vi "Intan_StreamData_128ch_parallelLoop.vi"(0 "VISA resource name":refnum<visa-resource-name>, 1 "refnum in":refnum<file>, 2 "NchansInStream":u16, 3 "stop streaming":bool, 4 "Save Binary Data":bool, 5 "error in":errorcluster, 7 "byte order":T5(ring)=enum."little-endian", 8 "hdr fpath":path, 9 "MaxStreamChans":u16=32, 11 "DT_scale (sec)":dbl=0.01, 12 "aux file ref num":refnum<file>, 14 "save aux file":bool) -> (6 "N data scans to read (VISA)":i32=20, 10 "Nbytes VISA read":u32, 13 "VISA read iter":i32, 19 "error out":errorcluster)   [LabVIEW 2017]
doc: "Stream data to disk and user friendly display. Data is scaled and filtered prior to display.\n\nThis VI uses parallel while loop architecture: 1 loop reads from serial stream and saves raw bytes to disk; the other loop processes the data in chunk, scaling and filtering, then displays."
uses:
  zip_swcircularbuffer1_0_19b/Circular Buffer/Controls/Circular Buffer Status.ctl
  zip_swcircularbuffer1_0_19b/Circular Buffer/Controls/Circular Buffer Operations.ctl
  <vilib>/Utility/error.llb/DialogType.ctl
  zip_swcircularbuffer1_0_19b/Circular Buffer/Instance VIs/Circular Buffer(1D U16).vi
  zip_swcircularbuffer1_0_19b/Circular Buffer/Circular Buffer.lvlib
panel:
  out "bytesParsed":i32=148
  out "Buffer Status Empty Buf":T1
  out "termcharsReadBuffer":string
  out "termcharsCount":u32
  out "NumChansNewStream":string
  out "Data Out":u16[](array[numeric])
  out "Elements Remaining":i32
  out "ChanSelString":string
  out "ChanSelect(uint32)":u32[](array[numeric])
  out "A+B+C+D chans":i32[](array[numeric])
  out "C+D chans":i32[](array[numeric])
  out "Dchans":i32[](array[numeric])
  out "Cchans":i32[](array[numeric])
  out "ADXL Stream":dbl[][](graph)
  out "A+B chans":i32[](array[numeric])
  out "Bchans":i32[](array[numeric])
  out "Achans":i32[](array[numeric])
  in  "Tab Control":T2(tab)
  in  "Update Channels":bool
  in  "Accel/Vbat":i32[](listbox)
  in  "stop logging":bool
  in  "DisplayScale (uV/div)":u16(ring)=1 items=["6400", "3200", "1600", "800", "400", "200", "100", "50", "25"]
  in  "offset factor":dbl=1.0
  in  "Filter settings":T3={"LP Filter On/Off"=TRUE, "LP Cutoff (Hz)"=40.0, "HP Filter On/Off"=TRUE, "HP Cutoff (Hz)"=0.5, "Bandstop On/Off"=TRUE, "fl Cutoff (Hz)"=48.0, "fh Cutoff (Hz) "=52.0}
  out "Save status":bool
  out "non integer read":bool
  out "display iter":i32
  out "% buffer full":dbl(slide) scale=0.0..100.0
  in  "Ring Buffer Size":T4={"Samples per Channel"=640000, "Channels"=0}
  out "buffer underflow":bool
  out "Buffer Status  (read)":T1
  out "buffer overflow":bool
  out "Buffer Status (write)":T1
  in  "Center Traces":bool
  in  "Amplifier Chans":i32[](listbox)=[1, 4, 13, 14, 15, 16, 17, 22]
  out "FS (Hz)":dbl
  in  "ChartDisplayLength (s)":dbl=5.0
  in  "Display Update interval (ms)":dbl=100.0
  in  "Buffer Read Interval (ms)":dbl=100.0
  in  "ChanSelect":u16(ring) items=["A chans (0-31)", "B chans (32-63)", "C chans (64-95)", "D chans (96-127)", "Free Select"]
  in  "bytes per data frame":i32=286
  in  "Nchans":i32=128
  in  "start stream (Teensy char)":string="s"
  in  "stop serial stream (Teensy char)":string="t"
  out "Text response":string
  out "timestamp_array":i32[](array[numeric])
  out "aux_cmd_array":i32[][](array[numeric])
  out "binary data (from VISA read)":u16[](array[numeric])
  out "magicNum Out":i32[](array[numeric])
  in  "stop logging Teensy char":string="l"
  out "Vdd (V) out":dbl[](array[numeric])
  out "setscaleresult":dbl
  out "UpdateCode":i16
  out "xmax_init":dbl
  out "offset_init":dbl
  out "increment_init":dbl
  out "xmin_init":dbl
  out "NchansChanged":bool
  out "DispLengthChanged":bool
  out "XscaleRollover":bool
  out "error code out":i32 format="%0.0f"
  out "StopLoopsMaster":bool
  out "N_u16s  write to buf":i32
  out "Nelements to read from buf":dbl
  out "N data scans to display":u16=20
  out "YtxtLabelsAll":string[](array[string])
  out "bytes streaming per frame":u16
  out "requestBytes":dbl
  out "SerRead":string
  out "Picture":picture
  out "Intan Streaming Data":dbl[][](graph)
  # "Intan-Teensy Bioelectric Module: Data Stream and Visualization\n128 chan + ADXL"
  # "Data Streaming Frequency"
  # "Display Settings"
  # "Ring Buffer Status"
  # "1-D data stream \nreformatted  to 2-D"
  # "xscale controls"
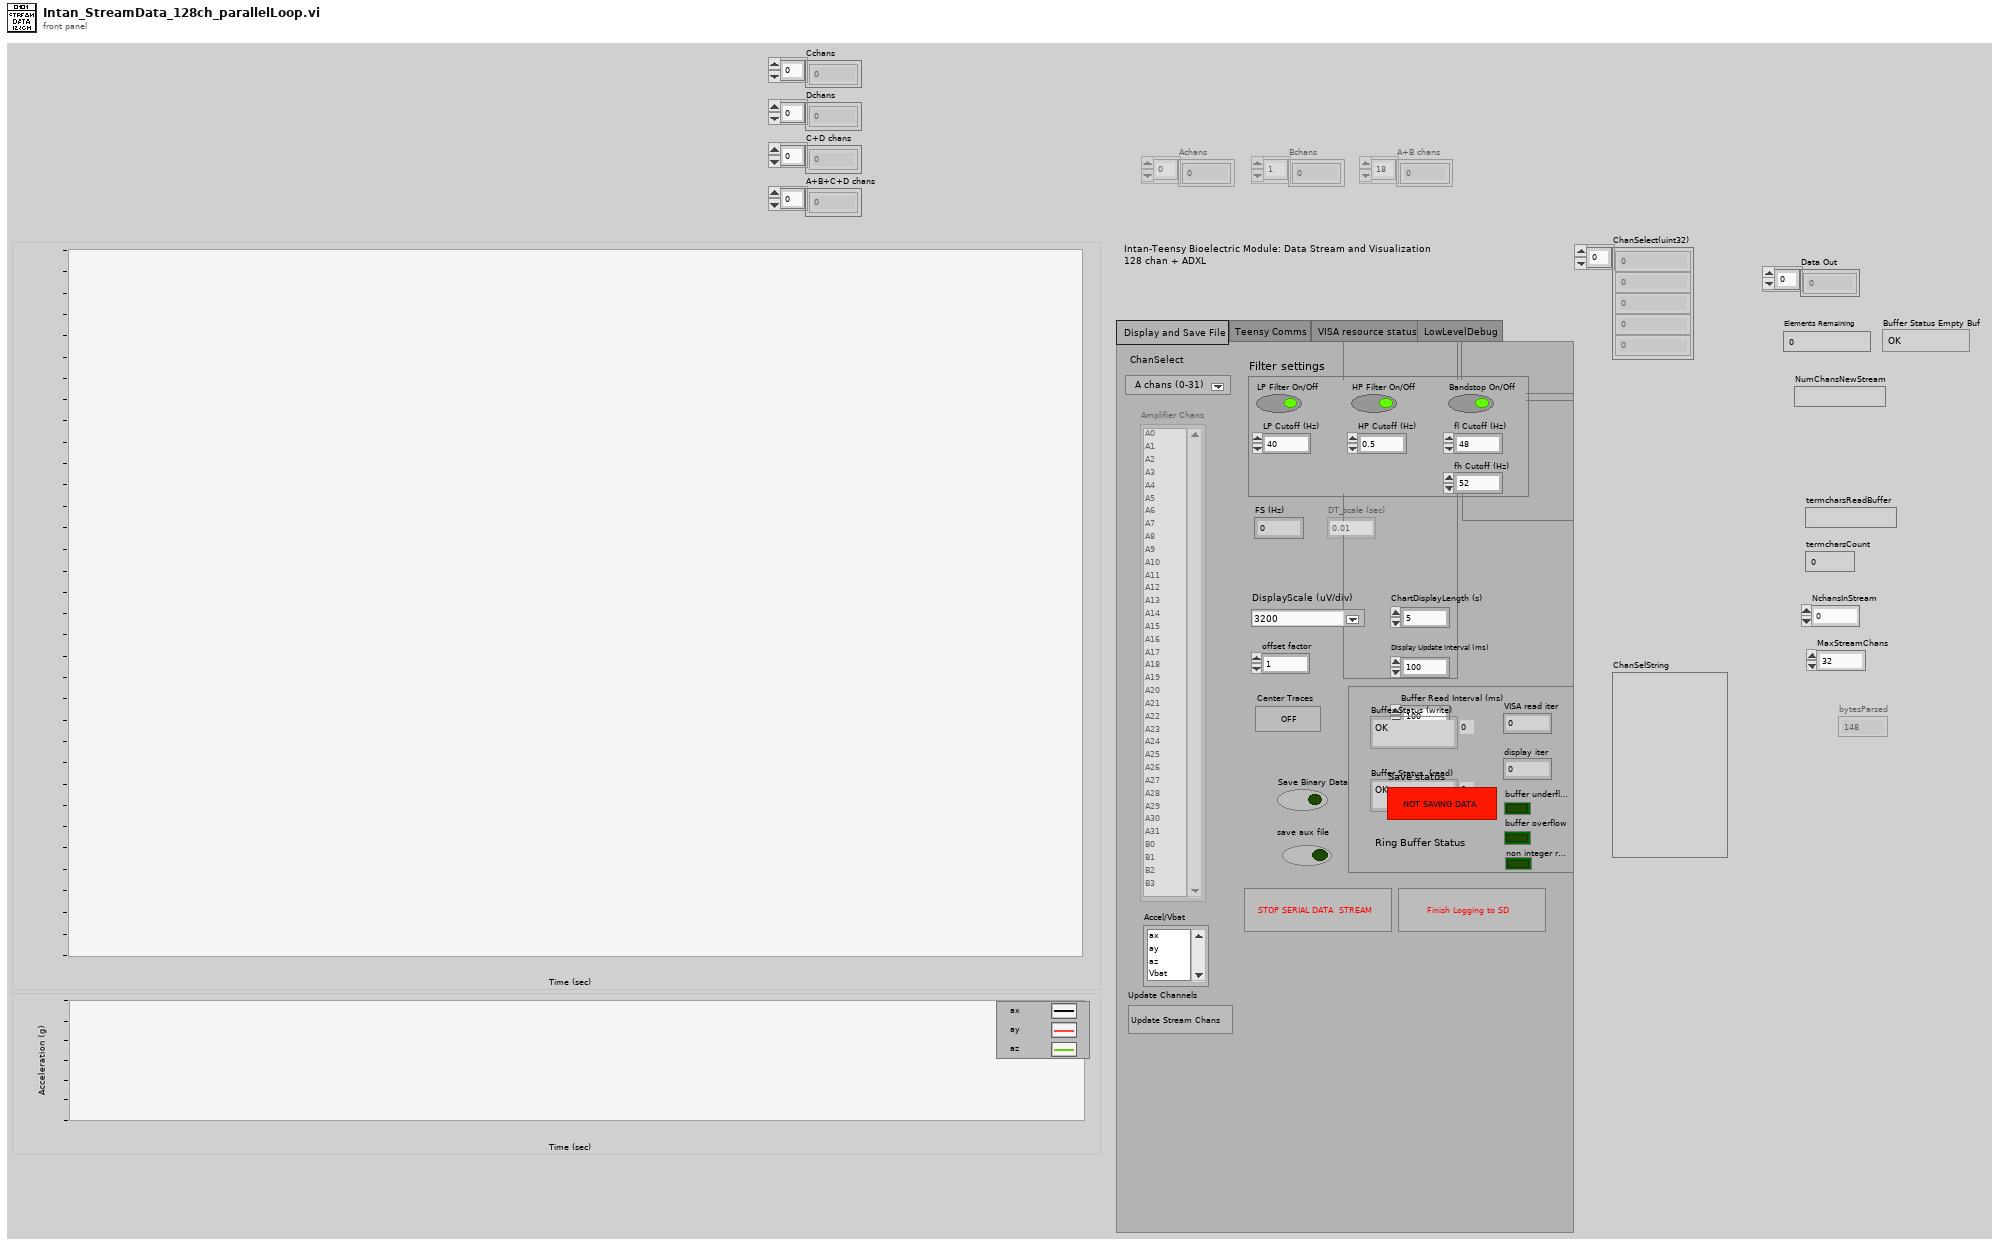
[diagram p1: front panel]
types:
  T1 = typedef "Circular Buffer.lvlib/Circular Buffer Status.ctl" = enum16{"OK", "Overflow", "Underflow"}
  T2 = enum32{"Display and Save File ", "Teensy Comms", "VISA resource status", "LowLevelDebug"}
  T3 = cluster{"LP Filter On/Off":bool, "LP Cutoff (Hz)":dbl, "HP Filter On/Off":bool, "HP Cutoff (Hz)":dbl, "Bandstop On/Off":bool, "fl Cutoff (Hz)":dbl, "fh Cutoff (Hz) ":dbl}
  T4 = cluster{"Samples per Channel":u32, "Channels":u32}
  T5 = enum16{"big-endian, network order", "native, host order", "little-endian"}
  T6 = typedef "Circular Buffer.lvlib/Circular Buffer Operations.ctl" = enum16{"Initialize", "Get Backlog", "Write", "Read (continuous)", "Read (most recent)"}
  T7 = enum8{"Enabled", "Disabled", "Disabled and Grayed Out"}
  T8 = typedef "LVRectTypeDef.ctl" = cluster{"Left":i16, "Top":i16, "Right":i16, "Bottom":i16}
  T9 = cluster{"XScale.Minimum":dbl, "XScale.Maximum":dbl, "XScale.Increment":dbl, "Nchannels":i32}
  T10 = cluster{"Maximum":dbl, dbl, dbl, dbl, dbl, dbl, "YscleMark":dbl, "Increment":dbl}
  T11 = typedef "DialogType.ctl" = u16
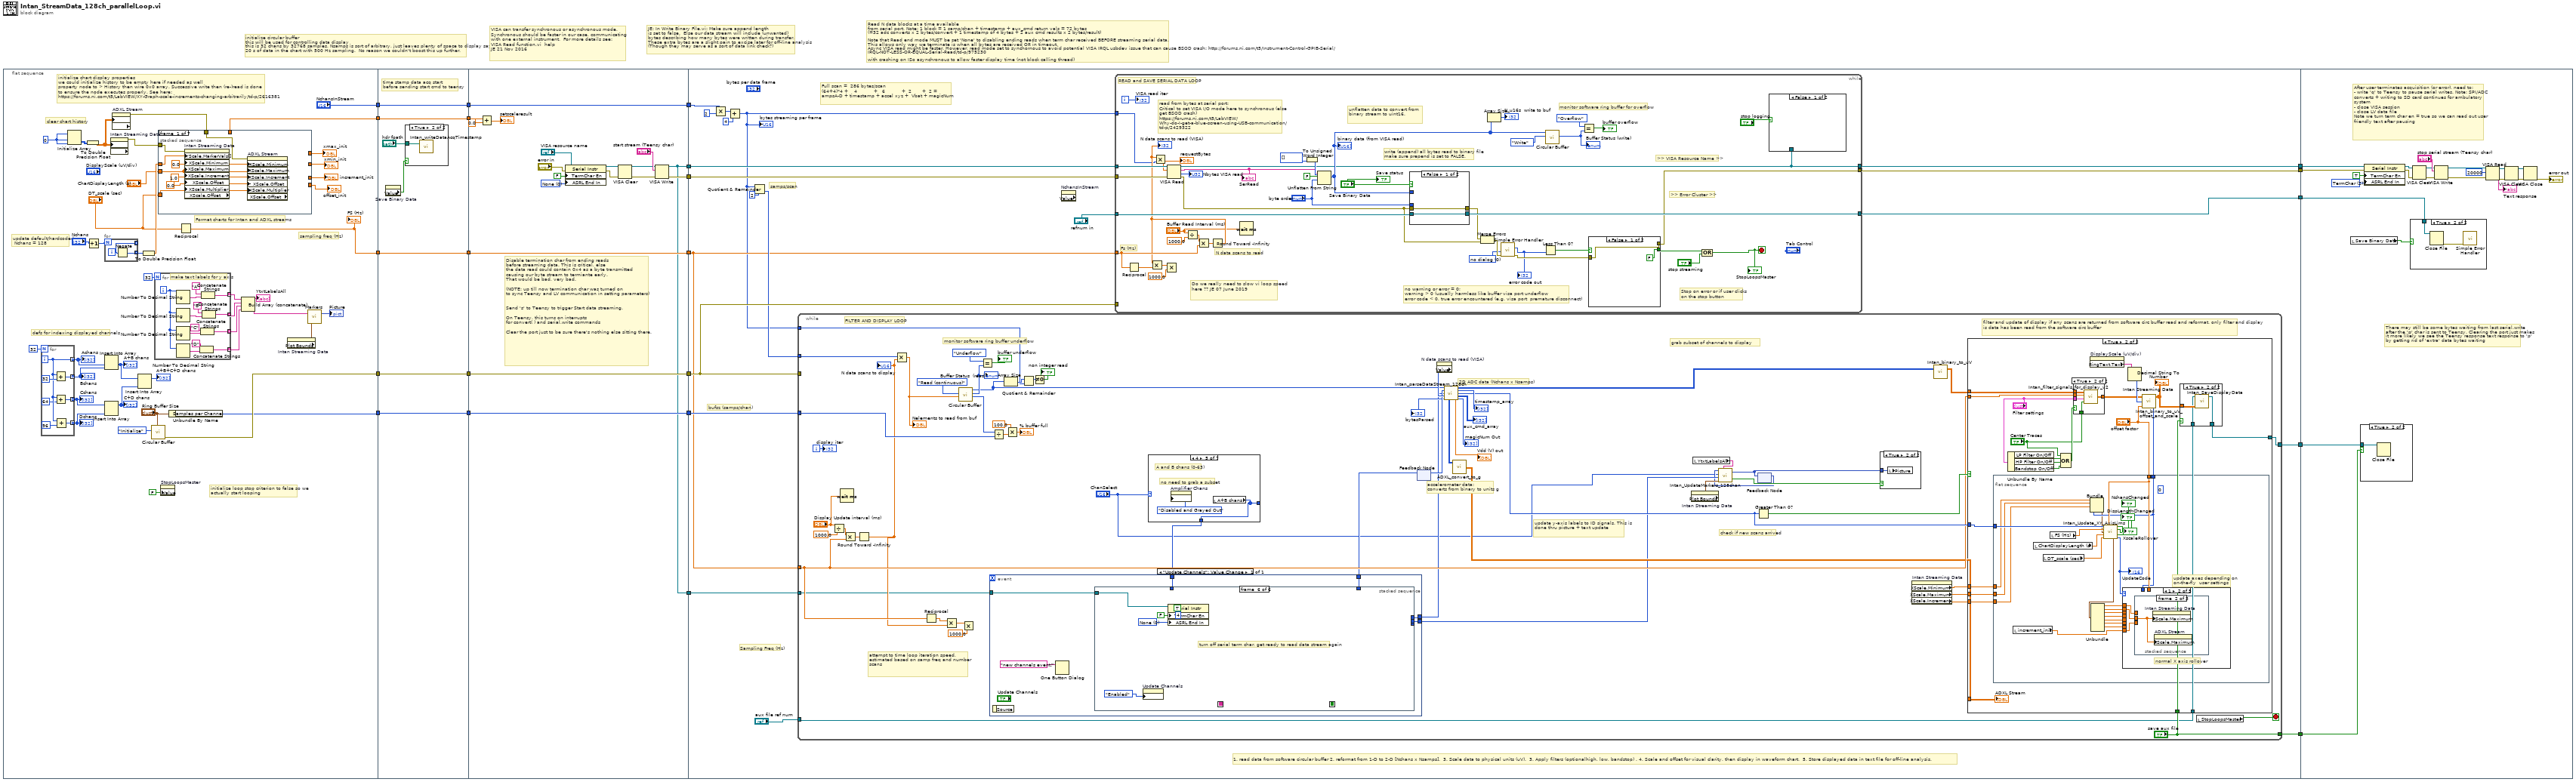
[diagram p0: block diagram]
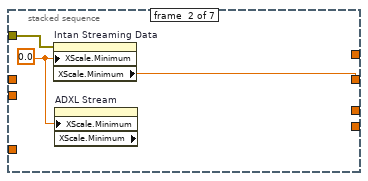
[diagram p2: hidden frame]
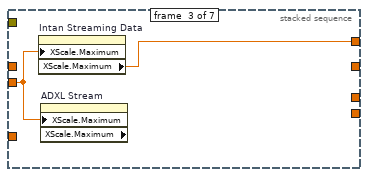
[diagram p3: hidden frame]
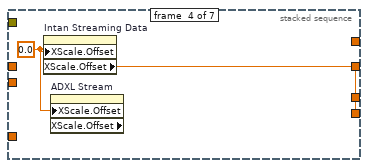
[diagram p4: hidden frame]
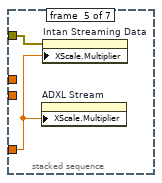
[diagram p5: hidden frame]
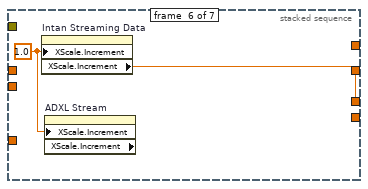
[diagram p6: hidden frame]
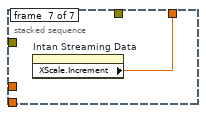
[diagram p7: hidden frame]
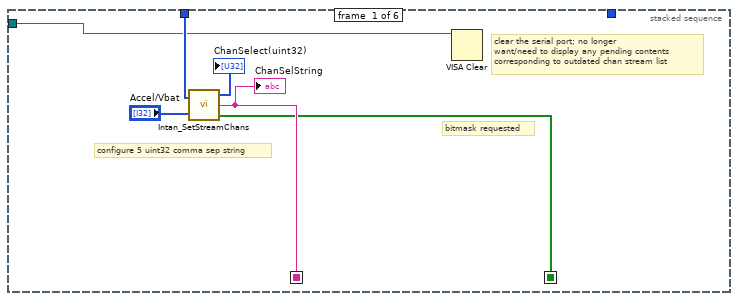
[diagram p9: hidden frame]
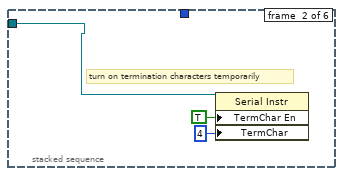
[diagram p10: hidden frame]
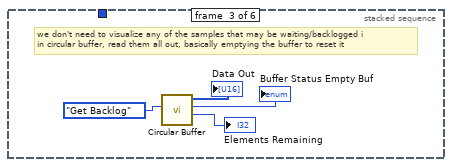
[diagram p11: hidden frame]
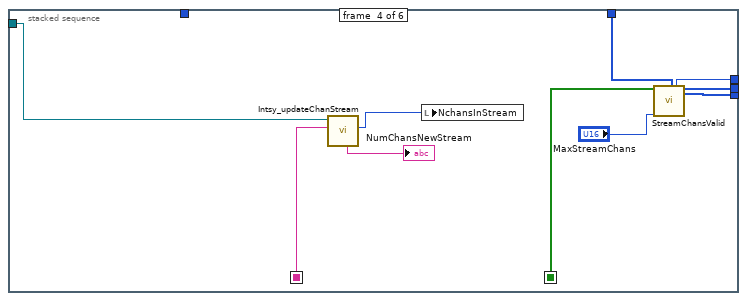
[diagram p12: hidden frame]
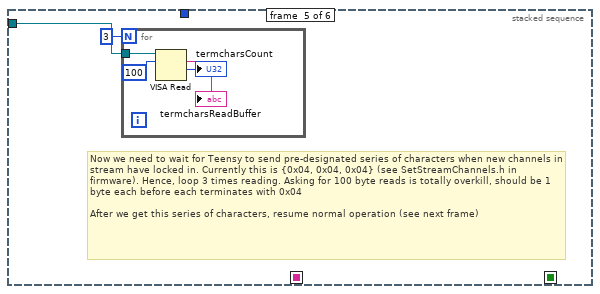
[diagram p13: hidden frame]
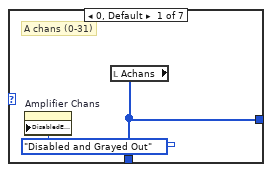
[diagram p15: hidden frame]
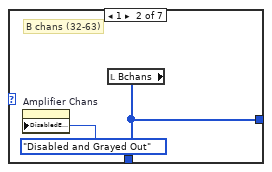
[diagram p16: hidden frame]
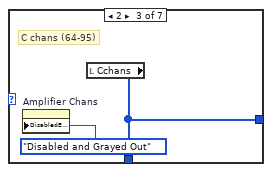
[diagram p17: hidden frame]
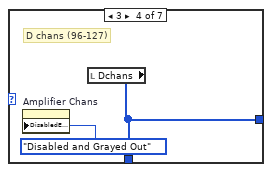
[diagram p18: hidden frame]
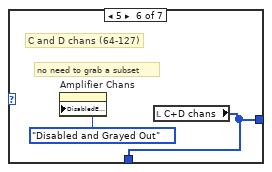
[diagram p19: hidden frame]
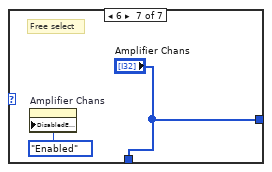
[diagram p20: hidden frame]
diagram:
  # "Read N data blocks at a time available\nfrom serial port. Note: 1 block = 1 samp/chan + timestamp + aux_cmd return vals = 72 bytes \n(=32 adc converts x 2 bytes/convert + 1 timestamp of 4 bytes + 2 aux cmd results x 2 bytes/result) \n\nNote that Read end mode MUST be set 'None' to disabling ending reads when term char received BEFORE streaming serial data.  \nThis allows only way we terminate is when all bytes are received OR in timeout.  \nAsync VISA read might be faster. However, read mode set to synchornous to avoid potential VISA IRQL usbdev issue that can cause BSOD crash: http://forums.ni.com/t5/Instrument-Control-GPIB-Serial/IRQL-NOT-LESS-OR-EQUAL-Serial-Read/td-p/975230\n\nwith crashing on ISo asynchronous to allow faster display time (not block calling thread)"
  # "initialize circular buffer\nthis will be used for controlling data display\nthis is 32 chans by 32768 samples. Nsamps is sort of arbitrary, just leaves plenty of space to display say\n20 s of data in the chart with 500 Hz sampling.  No reason we couldn't boost this up further."
  # "JE: In Write Binary File.vi: Make sure append length \nis set to false.  Else our data stream will include (unwanted)\nbytes describing how many bytes were written during transfer.\nThese extra bytes are a slight pain to excise later for off-line analysis\n(Though they may serve as a sort of data link check?)"
  # "VISA can transfer synchronous or asynchronous mode.\nSynchronous should be faster in our case, communicating\nwith one external instrument.  For more details see: \nVISA Read function.vi  help \nJE 21 Nov 2016"
  n1 = flat-sequence {
    tunnel: [w58] -> w12
    tunnel: [w56] -> w10
    tunnel: [w52] -> w8
    tunnel: [w41] -> w6
    tunnel: ["NchansInStream"] -> w3
    tunnel: w12 -> [w110]
    tunnel: [w110] -> w11
    tunnel: w10 -> [w109]
    tunnel: [w109] -> w9
    tunnel: w8 -> [w108]
    tunnel: [w108] -> w7
    tunnel: w6 -> [w107]
    tunnel: [w107] -> w5
    tunnel: w3 -> [w104]
    tunnel: [w104] -> w1
    tunnel: [w120] -> w20
    tunnel: [w113] -> w19
    tunnel: [w119] -> w18
    tunnel: w11 -> [w119]
    tunnel: [w118] -> w17
    tunnel: w9 -> [w118]
    tunnel: [w117] -> w16
    tunnel: w7 -> [w117]
    tunnel: w5 -> [w116]
    tunnel: [w113] -> w4
    tunnel: [w112] -> w2
    tunnel: w1 -> [w112]
    tunnel: [w145] -> w22
    tunnel: [w148] -> w21
    tunnel: w20 -> [w146]
    tunnel: w19 -> [w147]
    tunnel: w18 -> [w144]
    tunnel: w17 -> [w142]
    tunnel: w16 -> [w140]
    tunnel: [w139] -> w15
    tunnel: [w137] -> w14
    tunnel: [w136] -> w13
    tunnel: w4 -> [w135]
    tunnel: w2 -> [w134]
    tunnel: w22 -> [w425]
    tunnel: w21 -> [w438]
    tunnel: w15 -> [w420]
    tunnel: w14 -> [w419]
    tunnel: w13 -> [w418]
    frame #0 {
      w51 = 0 ("Dimension Size")
      # "Format charts for Intan and ADXL streams"
      # "defs for indexing displayed channels"
      # "update default/hardcoded\n Nchans = 128"
      # "clear chart history"
      # "initialize loop stop criterion to false so we\nactually start looping"
      # "sampling freq (Hz)"
      # "initialize chart display properties\nwe could initialize history to be empty here if needed as well\nproperty node to > History then wire 0x0 array. Successive write then (re-)read is done\nto ensure the node executes properly. See here:\nhttps://forums.ni.com/t5/LabVIEW/XY-Graph-scale-increments-changing-arbitrarily/td-p/2616381"
      n2 = for {
        N: 32 -> [_]
        tunnel: [w66] -> w33 mode=indexing
        tunnel: [w67] -> w32 mode=indexing
        tunnel: [w63] -> w31 mode=indexing
        tunnel: [w62] -> w30 mode=indexing
        i -> [w66]
        n3 = Add(x=w66, y=32) -> (x+y=w67:i32)
        n4 = Add(x=w66, y=64) -> (x+y=w63:i32)
        n5 = Add(x=w66, y=96) -> (x+y=w62:i32)
      }
      "Achans" <- w33
      "Bchans" <- w32
      "Cchans" <- w31
      "Dchans" <- w30
      n6 = Initialize Array(w51, w51, w51) -> (w50:i32[][])
      n7 = To Double Precision Float(number=w50) -> (double precision float=w35:dbl[][])
      n8 = Increment(x="Nchans") -> (x+1=w60:i32)
      n9 = for {
        N: w60 -> [_]
        tunnel: [w103] -> w61 mode=indexing
        tunnel: [w102] -> _ mode=indexing
        i -> [w102]
        n10 = Negate(x=w102) -> (-x=w103:i32)
      }
      n11 = Insert Into Array(array=w33, new element=w32) -> (w29:i32[])  [unwired: 1 in]
      "A+B chans" <- w29
      n12 = Insert Into Array(array=w31, new element=w30) -> (w28:i32[])  [unwired: 1 in]
      "C+D chans" <- w28
      n13 = property on="Intan Streaming Data" class="WFChart (strict)" props=["History Data", "History Data"]("History Data"=w35) -> (error out=w48:errorcluster)  [unwired: 2 in, 2 out]
      n14 = property on="ADXL Stream" class="WFChart (strict)" props=["History Data", "History Data"]("History Data"=w35) -> (error out=w34:errorcluster)  [unwired: 2 in, 2 out]
      n15 = Insert Into Array(array=w29, new element=w28) -> (→"A+B+C+D chans":i32[])  [unwired: 1 in]
      n16 = To Double Precision Float(number=w61) -> (double precision float=w49:dbl[])
      n17 = call-poly "Circular Buffer.vi"("Buffer Size"="Ring Buffer Size", "Operation"=Circular_Buffer_Operations."Initialize") -> ("error out"=w58:errorcluster)  [unwired: 6 in, 3 out]
      n18 = for {
        N: 32 -> [_]
        tunnel: [w99] -> w38 mode=indexing
        tunnel: [w96] -> w37 mode=indexing
        tunnel: [w90] -> w26 mode=indexing
        tunnel: [w89] -> w25 mode=indexing
        i -> [w95]
        # "make text labels for y axis"
        n19 = Number To Decimal String(number=w95) -> (decimal integer string=w101:string)  [unwired: 1 in]
        n20 = Number To Decimal String(number=w95) -> (decimal integer string=w98:string)  [unwired: 1 in]
        n21 = Number To Decimal String(number=w95) -> (decimal integer string=w91:string)  [unwired: 1 in]
        n22 = Number To Decimal String(number=w95) -> (decimal integer string=w92:string)  [unwired: 1 in]
        n23 = Concatenate Strings("D" ("string"), w92) -> (w89:string)
        n24 = Concatenate Strings("C" ("string"), w91) -> (w90:string)
        n25 = Concatenate Strings("A" ("string"), w101) -> (w99:string)
        n26 = Concatenate Strings("B" ("string"), w98) -> (w96:string)
      }
      n27 = stacked-sequence {
        tunnel: w49 -> [w76 _ _ _ _ _ _]
        tunnel: w48 -> [w75 w78 _ _ w85 _ _]
        tunnel: "ChartDisplayLength (s)" -> [w73 _ w80 _ _ _ _]
        tunnel: "DT_scale (sec)" -> [w70 _ _ _ w84 _ _]
        tunnel: [_ _ w81 _ _ _ _] -> w42
        tunnel: [_ w79 _ _ _ _ _] -> w45
        tunnel: [_ _ _ _ _ w87 _] -> w44
        tunnel: [_ _ _ w83 _ _ _] -> w43
        tunnel: [_ _ _ _ _ _ w88] -> w41
        tunnel: w34 -> [w69 _ _ _ _ _ _]
        frame #0 {
          w72 = 1.0 ("X Scale.Range:Minimum")
          w71 = 0.0 ("X Scale.Range:Minimum")
          w74 = 0.0 ("X Scale.Range:Minimum")
          n28 = property on="Intan Streaming Data" class="WFChart (strict)" props=["YScale", "MarkerVals[]", "XScale", "Minimum", "XScale", "Maximum", "XScale", "Increment", "XScale", "Offset", "XScale", "Multiplier", "XScale", "Offset"](error in=w75, "YScale.MarkerVals[]"=w76, "XScale.Minimum"=w74, "XScale.Maximum"=w73, "XScale.Increment"=w72, "XScale.Offset"=w71, "XScale.Multiplier"=w70) -> ()  [unwired: 1 in, 3 out]
          n29 = property on="ADXL Stream" class="WFChart (strict)" props=["XScale", "Minimum", "XScale", "Maximum", "XScale", "Increment", "XScale", "Offset", "XScale", "Multiplier", "XScale", "Offset"](error in=w69, "XScale.Minimum"=w74, "XScale.Maximum"=w73, "XScale.Increment"=w72, "XScale.Offset"=w71, "XScale.Multiplier"=w70) -> ()  [unwired: 1 in, 3 out]
        }
        frame #1 {
          w77 = 0.0 ("X Scale.Range:Minimum")
          n30 = property on="Intan Streaming Data" class="WFChart (strict)"(error in=w78, "XScale.Minimum"=w77) -> ("XScale.Minimum"=w79:dbl)  [unwired: 1 in, 2 out]
          n31 = property on="ADXL Stream" class="WFChart (strict)" props=["XScale", "Minimum", "XScale", "Minimum"]("XScale.Minimum"=w77) -> ()  [unwired: 2 in, 3 out]
        }
        frame #2 {
          n32 = property on="Intan Streaming Data" class="WFChart (strict)"("XScale.Maximum"=w80) -> ("XScale.Maximum"=w81:dbl)  [unwired: 2 in, 2 out]
          n33 = property on="ADXL Stream" class="WFChart (strict)" props=["XScale", "Maximum", "XScale", "Maximum"]("XScale.Maximum"=w80) -> ()  [unwired: 2 in, 3 out]
        }
        frame #3 {
          w82 = 0.0 ("X Scale.Offset and Multiplier:Offset")
          n34 = property on="Intan Streaming Data" class="WFChart (strict)"("XScale.Offset"=w82) -> ("XScale.Offset"=w83:dbl)  [unwired: 2 in, 2 out]
          n35 = property on="ADXL Stream" class="WFChart (strict)" props=["XScale", "Offset", "XScale", "Offset"]("XScale.Offset"=w82) -> ()  [unwired: 2 in, 3 out]
        }
        frame #4 {
          n36 = property on="ADXL Stream" class="WFChart (strict)"("XScale.Multiplier"=w84) -> ()  [unwired: 2 in, 2 out]
          n37 = property on="Intan Streaming Data" class="WFChart (strict)"(error in=w85, "XScale.Multiplier"=w84) -> ()  [unwired: 1 in, 2 out]
        }
        frame #5 {
          w86 = 1.0 ("X Scale.Range:Increment")
          n38 = property on="Intan Streaming Data" class="WFChart (strict)"("XScale.Increment"=w86) -> ("XScale.Increment"=w87:dbl)  [unwired: 2 in, 2 out]
          n39 = property on="ADXL Stream" class="WFChart (strict)" props=["XScale", "Increment", "XScale", "Increment"]("XScale.Increment"=w86) -> ()  [unwired: 2 in, 3 out]
        }
        frame #6 {
          n40 = property on="Intan Streaming Data" class="WFChart (strict)"() -> ("XScale.Increment"=w88:dbl)  [unwired: 2 in, 2 out]
        }
      }
      "xmin_init" <- w45
      "increment_init" <- w44
      "offset_init" <- w43
      "xmax_init" <- w42
      n41 = property on="StopLoopsMaster" class="Bool (strict)"("Value"=FALSE ("StopLoopsMaster")) -> ()  [unwired: 2 in, 2 out]
      n42 = Unbundle By Name("Ring Buffer Size") -> ("Samples per Channel"=w56:u32)
      n43 = Reciprocal(x="DT_scale (sec)") -> (1/x=w52:dbl)
      "FS (Hz)" <- w52
      n44 = Build Array (concatenate)(w38, w37, w26, w25) -> (w36:string[])
      "YtxtLabelsAll" <- w36
      n45 = property on="Intan Streaming Data" class="WFChart (strict)"() -> ("Plot Bounds"=w53:T8)  [unwired: 2 in, 2 out]
      n46 = call "Markers.vi"("plot bounds"=w53, "Array"=w36) -> ("Picture"=→"Picture":picture)  [unwired: 1 out]
    }
    frame #1 {
      # "time stamp data acq start\nbefore sending start cmd to teensy"
      n47 = property on="Save Binary Data" class="Bool (strict)"() -> ("Value"=w106:bool)  [unwired: 2 in, 2 out]
      n48 = case shown="True" w106 {
        tunnel: "hdr fpath" -> [_ w111]
        frame False {
        }
        frame True {
          n49 = call "Intan_writeDataAcqTimestamp.vi"("hdr fpath"=w111) -> ()  [unwired: 2 in, 1 out]
        }
      }
    }
    frame #2 {
      w125 = u16 0 items=["None", "Last Bit", "TermChar"] ("Serial Settings:End Mode for Reads")
      # "Disable termination char from ending reads\nbefore streaming data. This is critical, else\nthe data read could contain 0x4 as a byte transmitted\ncausing our byte stream to termiante early.\nThat would be bad, very bad.\n\n(NOTE: up till now termination char was turned on\nto sync Teensy and LV communication in setting parameters)\n\n\nSend 's' to Teensy to trigger Start data streaming.  \n\nOn Teensy, this turns on interrupts\nfor convert( ) and serial.write commands\n\nClear the port just to be sure there's nothing else sitting there."
      n50 = Add(x=w116, y=0.0) -> (x+y=→"setscaleresult":dbl)
      n51 = property class="Serial Instr"(reference="VISA resource name", error in="error in", "TermChar En"=FALSE ("Message Based Settings:Termination Character Enable"), "ASRL End In"=w125) -> (reference out=w124:refnum<visa-resource-name>, error out=w123:errorcluster)
      n52 = VISA Clear(VISA resource name=w124, error in (no error)=w123) -> (VISA resource name out=w122:refnum<visa-resource-name>, error out=w121:errorcluster)
      n53 = VISA Write(VISA resource name=w122, write buffer="start stream (Teensy char)", error in (no error)=w121) -> (VISA resource name out=w113:refnum<visa-resource-name>, error out=w120:errorcluster)  [unwired: 1 out]
    }
    frame #3 {
      # "Full scan =  286 bytes/scan\n(64+4)*4 +    4           +   6           +  2       +  2 =\nampsA-D + timestamp + accel xyz +  Vbat + magicNum"
      # "1. read data from software circular buffer 2. reformat from 1-D to 2-D [Nchans x Nsamps].  3. Scale data to physical units (uV).  3. Apply filters (optionalhigh, low, bandstop) . 4. Scale and offset for visual clarity, then display in waveform chart.  5. Store displayed data in text file for off-line analysis."
      # "Sampling Freq (Hz)"
      # "bufsz (samps/chan)"
      # "samps/scan"
      n54 = Multiply(x=w134, y=u16 2) -> (x*y=w132:u16)
      n55 = Add(x=w132, y=u16 4) -> (x+y=w130:u16)
      "bytes streaming per frame" <- w130
      n56 = Quotient & Remainder(x=w130, y=i16 2) -> (floor(x/y)=w141:u16)  [unwired: 1 out]
      n57 = while {
        tunnel: w144 -> [_]
        tunnel: w142 -> [w201]
        tunnel: w140 -> [w173]
        tunnel: w141 -> [w194]
        tunnel: [w178] -> w139
        tunnel: "aux file ref num" -> [w177]
        tunnel: ["save aux file"] -> w136
        tunnel: w135 -> [w160]
        tunnel: w130 -> [w150]
        i -> [w195]
        stop <- w175 stop-if-true
        # "accelerometer data: \nconverts from binary to units g"
        # "2D ADC data (Nchans x Nsamps)"
        # "check if new scans arrived"
        # "grab subset of channels to display"
        # "update y-axis labels to ID signals. This is done thru picture + text update"
        # "FILTER AND DISPLAY LOOP"
        # "attempt to time loop iteration speed,\nestimated based on samp freq and number scans"
        # "filter and update of display if any scans are returned from software circ buffer read and reformat. only filter and display is data has been read from the software circ buffer"
        # "monitor software ring buffer underflow"
        n58 = Divide(x="Display Update interval (ms)", y=1000.0) -> (x/y=w170:dbl)
        n59 = Wait (ms)(milliseconds to wait="Display Update interval (ms)") -> ()  [unwired: 1 out]
        n60 = Multiply(x=w170, y=w173) -> (x*y=w172:dbl)
        n61 = Round Toward -Infinity(1:w172) -> (0:w171:dbl)
        "N data scans to display" <- w171
        n62 = Multiply(x=w194, y=w171) -> (x*y=w193:dbl)
        "Nelements to read from buf" <- w193
        n63 = Reciprocal(x=w173) -> (1/x=w186:dbl)
        n64 = Multiply(x=w186, y=w171) -> (x*y=w185:dbl)
        n65 = call-poly "Circular Buffer.vi"("Read Size"=w193, "Operation"=Circular_Buffer_Operations."Read (continuous)") -> ("Elements Remaining"=w202:i32, "Buffer Status"=w204:T1, "Data Out"=w190:u16[])  [unwired: 6 in, 1 out]
        "Buffer Status  (read)" <- w204
        n66 = Multiply(x=w185, y=1000.0) -> ()  [unwired: 1 out]
        n67 = Equal?(x=Circular_Buffer_Status."Underflow" ("y"), y=w204) -> (x = y?=→"buffer underflow":bool)
        n68 = Divide(x=w202, y=w201) -> (x/y=w200:dbl)
        n69 = Array Size(array=w190) -> (size(s)=w189:i32)
        n70 = Multiply(x=100.0, y=w200) -> (x*y=→"% buffer full":dbl)
        n71 = Quotient & Remainder(x=w189, y=w150) -> (x-y*floor(x/y)=w188:i32)  [unwired: 1 out]
        n72 = Not Equal To 0?(x=w188) -> (x != 0?=→"non integer read":bool)
        n73 = case shown="4" "ChanSelect" {
          tunnel: [w246 w248 w250 w252 w254 w256 "Amplifier Chans"] -> _
          tunnel: [w246 w248 w250 w252 w254 w256 "Amplifier Chans"] -> w161
          frame 0, Default {
            # "A chans (0-31)"
            n74 = property on="Amplifier Chans" class="LstBox (strict)"("DisabledEnum"=T7."Disabled and Grayed Out" ("Disabled")) -> ()  [unwired: 2 in, 2 out]
            n75 = local read "Achans"() -> (w246:i32[])
          }
          frame 1 {
            # "B chans (32-63)"
            n76 = property on="Amplifier Chans" class="LstBox (strict)"("DisabledEnum"=T7."Disabled and Grayed Out" ("Disabled")) -> ()  [unwired: 2 in, 2 out]
            n77 = local read "Bchans"() -> (w248:i32[])
          }
          frame 2 {
            # "C chans (64-95)"
            n78 = property on="Amplifier Chans" class="LstBox (strict)"("DisabledEnum"=T7."Disabled and Grayed Out" ("Disabled")) -> ()  [unwired: 2 in, 2 out]
            n79 = local read "Cchans"() -> (w250:i32[])
          }
          frame 3 {
            # "D chans (96-127)"
            n80 = property on="Amplifier Chans" class="LstBox (strict)"("DisabledEnum"=T7."Disabled and Grayed Out" ("Disabled")) -> ()  [unwired: 2 in, 2 out]
            n81 = local read "Dchans"() -> (w252:i32[])
          }
          frame 4 {
            # "A and B chans (0-63)"
            # "no need to grab a subset"
            n82 = property on="Amplifier Chans" class="LstBox (strict)"("DisabledEnum"=T7."Disabled and Grayed Out" ("Disabled")) -> ()  [unwired: 2 in, 2 out]
            n83 = local read "A+B chans"() -> (w254:i32[])
          }
          frame 5 {
            # "C and D chans (64-127)"
            # "no need to grab a subset"
            n84 = property on="Amplifier Chans" class="LstBox (strict)"("DisabledEnum"=T7."Disabled and Grayed Out" ("Disabled")) -> ()  [unwired: 2 in, 2 out]
            n85 = local read "C+D chans"() -> (w256:i32[])
          }
          frame 6 {
            # "Free select"
            n86 = property on="Amplifier Chans" class="LstBox (strict)"("DisabledEnum"=T7."Enabled" ("Disabled")) -> ()  [unwired: 2 in, 2 out]
          }
        }
        n87 = event shown="[0] \"Update Channels\": Value Change" {
          selector: _ -> [_]
          dyn-events: _ -> [_]
          timeout: _ -> [_]
          tunnel: w161 -> [w212]
          tunnel: w160 -> [w210]
          tunnel: [w209] -> w159
          tunnel: [w208] -> w154
          tunnel: [w207] -> w153
          event "Update Channels": Value Change {
            n88 = event-data() -> ()  [unwired: 1 in, 1 out]
            n89 = One Button Dialog(message="new channels event!") -> ()  [unwired: 1 in, 1 out]
            n90 = stacked-sequence {
              seq-local: [w215 _ _ _ _ _] -> [_ _ _ w229 _ _]
              seq-local: [w213 _ _ _ _ _] -> [_ _ _ w234 _ _]
              tunnel: w212 -> [w217 _ _ _ _ _]
              tunnel: w210 -> [w216 w219 _ w228 w236 w242]
              tunnel: [_ _ _ w231 _ _] -> _
              tunnel: [_ _ _ w232 _ _] -> w208
              tunnel: [_ _ _ w231 _ _] -> w209
              tunnel: [_ _ _ w230 _ _] -> w207
              frame #0 {
                # "bitmask requested"
                # "clear the serial port; no longer\nwant/need to display any pending contents\ncorresponding to outdated chan stream list"
                # "configure 5 uint32 comma sep string"
                n91 = call "Intan_SetStreamChans.vi"("Amplifier Chans"=w217, "Accel/Vbat"="Accel/Vbat") -> ("ChanSelect(uint32)"=→"ChanSelect(uint32)":u32[], "ChanSelString"=w215:string, "BitMaskAll"=w213:bool[])
                "ChanSelString" <- w215
                n92 = VISA Clear(VISA resource name=w216) -> ()  [unwired: 1 in, 2 out]
              }
              frame #1 {
                # "turn on termination characters temporarily"
                n93 = property class="Serial Instr"(reference=w219, "TermChar En"=TRUE ("Message Based Settings:Termination Character Enable"), "TermChar"=u8 4 ("Message Based Settings:Termination Character")) -> ()  [unwired: 1 in, 2 out]
              }
              frame #2 {
                # "we don't need to visualize any of the samples that may be waiting/backlogged i\nin circular buffer, read them all out, basically emptying the buffer to reset it"
                n94 = call-poly "Circular Buffer.vi"("Operation"=Circular_Buffer_Operations."Get Backlog") -> ("Elements Remaining"=→"Elements Remaining":i32, "Buffer Status"=→"Buffer Status Empty Buf":T1, "Data Out"=→"Data Out":u16[])  [unwired: 7 in, 1 out]
              }
              frame #3 {
                n95 = call "Intsy_updateChanStream.vi"("ChanSelString"=w229, "VISA resource name"=w228) -> ("NChansInStream"=w227:i32, "NStreamChansString"=→"NumChansNewStream":string)  [unwired: 5 in, 3 out]
                n96 = local write "NchansInStream"(w227) -> ()
                n97 = call "StreamChansValid.vi"("BitMaskRequested"=w234, "MaxStreamChans"="MaxStreamChans") -> ("bitMaskI16"=w231:i16[], "NumChansStreaming"=w232:i16, "AmpsList"=w230:u16[])  [unwired: 8 in, 7 out]
              }
              frame #4 {
                # "Now we need to wait for Teensy to send pre-designated series of characters when new channels in stream have locked in. Currently this is {0x04, 0x04, 0x04} (see SetStreamChannels.h in firmware). Hence, loop 3 times reading. Asking for 100 byte reads is totally overkill, should be 1 byte each before each terminates with 0x04\n\nAfter we get this series of characters, resume normal operation (see next frame)"
                n98 = for {
                  N: 3 -> [_]
                  tunnel: w236 -> [w240]
                  n99 = VISA Read(VISA resource name=w240, byte count=u32 100) -> (read buffer=→"termcharsReadBuffer":string, return count=→"termcharsCount":u32)  [unwired: 1 in, 2 out]
                }
              }
              frame #5 {
                w243 = u16 0 items=["None", "Last Bit", "TermChar"] ("Serial Settings:End Mode for Reads")
                (unwired) u8 4 ("Message Based Settings:Termination Character")
                (unwired) TRUE ("Message Based Settings:Termination Character Enable")
                # "turn off serial term char, get ready to read data stream again"
                n100 = property on="Update Channels" class="Bool (strict)"("DisabledEnum"=T7."Enabled" ("Disabled")) -> ()  [unwired: 2 in, 2 out]
                n101 = property class="Serial Instr"(reference=w242, "TermChar En"=FALSE ("Message Based Settings:Termination Character Enable"), "ASRL End In"=w243) -> ()  [unwired: 1 in, 2 out]
              }
            }
          }
        }
        n102 = feedback-in #1(w159) -> ()
        n103 = feedback #1() -> (w158:i16[])  [unwired: 1 in]
        n104 = property on="N data scans to read (VISA)" class="DigNum (strict)"() -> ("Value"=w192:i32)  [unwired: 2 in, 2 out]
        n105 = call "Intan_parseDataStream_128ch.vi"("1-D  data in"=w190, "bitMaskI16"=w158, "NumChansStreaming"=w154, "N data scans to read"=w192) -> ("2d ADCdata_array out_ampA_and_B"=w155:u16[][], "timestamp_array"=→"timestamp_array":i32[], "Nscans read"=w176:i32, "aux_cmd_array A"=→"aux_cmd_array":i16[][], "bytes parsed per scan"=→"bytesParsed":i32, "ADXL analog data out"=w164:u16[][], "Vdd (V) out"=→"Vdd (V) out":dbl[], "MagicNumOut"=→"magicNum Out":i32[])  [unwired: 2 in, 2 out]
        n106 = call "ADXL_convert_to_g.vi"("ADXL analog data out: Binary format"=w164) -> ("ADXL scaled (units of g)"=w163:dbl[][])  [unwired: 3 in]
        n107 = property on="Intan Streaming Data" class="WFChart (strict)"() -> ("Plot Bounds"=w182:T8)  [unwired: 2 in, 2 out]
        n108 = local read "YtxtLabelsAll"() -> (w174:string[])
        n109 = Greater Than 0?(x=w176) -> (x > 0?=w191:bool)
        n110 = feedback #2() -> (w152:picture)  [unwired: 1 in]
        n111 = call "Intan_UpdateMarkers_128chan.vi"("Picture In"=w152, "ChanSelectMode"="ChanSelect", "Display Chans"=w153, "plot bounds"=w182, "YtxtLabelsAll"=w174) -> ("Picture Out"=w180:picture, "update labels"=w181:bool)
        n112 = feedback-in #2(w180) -> ()
        n113 = case shown="True" w181 {
          tunnel: w180 -> [_ w245]
          frame False {
          }
          frame True {
            n114 = local write "Picture"(w245) -> ()
          }
        }
        n115 = property on="Intan Streaming Data" class="WFChart (strict)"() -> ("XScale.Minimum"=w167:dbl, "XScale.Maximum"=w166:dbl, "XScale.Increment"=w165:dbl)  [unwired: 2 in, 2 out]
        n116 = call "Intan_binary_to_uV.vi"("2d ADC binary data"=w155) -> ("Scaled Data (uV)"=w183:dbl[][])  [unwired: 2 in]
        n117 = case shown="True" w191 {
          tunnel: w173 -> [_ w281]
          tunnel: w183 -> [_ w279]
          tunnel: [w260 w272] -> w178
          tunnel: "save aux file" -> [_ w271]
          tunnel: w177 -> [w260 w270]
          tunnel: w176 -> [_ w268]
          tunnel: w167 -> [_ w264]
          tunnel: w166 -> [_ w263]
          tunnel: w165 -> [_ w262]
          tunnel: w163 -> [_ w261]
          frame False {
          }
          frame True {
            n118 = flat-sequence {
              tunnel: w268 -> [w303]
              tunnel: "offset factor" -> [w290]
              tunnel: w265 -> [w287]
              tunnel: w264 -> [w285]
              tunnel: w263 -> [w284]
              tunnel: w262 -> [w283]
              frame #0 {
                (unwired) 0 ("index")
                # "update axes depending on\non-the-fly  user settings"
                n119 = local read "increment_init"() -> (w289:dbl)
                n120 = local read "ChartDisplayLength (s)"() -> (w301:dbl)
                n121 = local read "DT_scale (sec)"() -> (w300:dbl)
                n122 = local read "FS (Hz)"() -> (w302:dbl)
                n123 = Bundle("XScale.Minimum"=w285, "XScale.Maximum"=w284, "XScale.Increment"=w283, "Nchannels"=w287) -> (w286:T9)  [unwired: 1 in]
                n124 = call "Intan_Update_XY_AxisLims.vi"("NscansRead"=w303, "offset factor"=w290, "FS (Hz)"=w302, "XscaleClusterCurrent"=w286, "DisplayLength(s)"=w301, "DT_scale (s)"=w300) -> ("XscaleRollover"=→"XscaleRollover":bool, "DispLengthChanged"=→"DispLengthChanged":bool, "NchansChanged"=→"NchansChanged":bool, "XYlims Update Cluster"=w298:T10, "UpdateCode"=w299:i16)  [unwired: 4 in, 1 out]
                "UpdateCode" <- w299
                n125 = Unbundle(w298) -> ("Maximum"=w295:dbl, w294:dbl, w292:dbl, w291:dbl, w297:dbl, w296:dbl, "YscleMark"=w293:dbl)  [unwired: 1 out]
                n126 = case shown="1" w299 {
                  tunnel: w287 -> [_ _ _ w323 w334]
                  tunnel: w297 -> [_ _ _ w318 _]
                  tunnel: w296 -> [_ _ _ w322 _]
                  tunnel: w295 -> [_ w308 _ _ w337]
                  tunnel: w294 -> [_ w307 _ _ w336]
                  tunnel: w293 -> [_ _ _ w321 w335]
                  tunnel: w292 -> [_ _ w313 _ _]
                  tunnel: w291 -> [_ _ w314 _ _]
                  tunnel: w290 -> [_ _ _ w320 w333]
                  tunnel: w289 -> [_ w306 w312 w319 w332]
                  frame 0, Default {
                    # "nothing to update"
                  }
                  frame 1 {
                    # "normal X axis rollover"
                    n127 = stacked-sequence {
                      tunnel: w308 -> [w309 _ _]
                      tunnel: w307 -> [_ w310 _]
                      tunnel: w306 -> [_ _ w311]
                      frame #0 {
                        n128 = property on="Intan Streaming Data" class="WFChart (strict)"("XScale.Minimum"=w309) -> ()  [unwired: 2 in, 2 out]
                        n129 = property on="ADXL Stream" class="WFChart (strict)"("XScale.Minimum"=w309) -> ()  [unwired: 2 in, 2 out]
                      }
                      frame #1 {
                        n130 = property on="Intan Streaming Data" class="WFChart (strict)"("XScale.Maximum"=w310) -> ()  [unwired: 2 in, 2 out]
                        n131 = property on="ADXL Stream" class="WFChart (strict)"("XScale.Maximum"=w310) -> ()  [unwired: 2 in, 2 out]
                      }
                      frame #2 {
                        n132 = property on="Intan Streaming Data" class="WFChart (strict)"("XScale.Increment"=w311) -> ()  [unwired: 2 in, 2 out]
                        n133 = property on="ADXL Stream" class="WFChart (strict)"("XScale.Increment"=w311) -> ()  [unwired: 2 in, 2 out]
                      }
                    }
                  }
                  frame 2 {
                    # "updated display length"
                    n134 = stacked-sequence {
                      tunnel: w312 -> [_ _ w317]
                      tunnel: w314 -> [_ w316 _]
                      tunnel: w313 -> [w315 _ _]
                      frame #0 {
                        n135 = property on="Intan Streaming Data" class="WFChart (strict)"("XScale.Minimum"=w315) -> ()  [unwired: 2 in, 2 out]
                        n136 = property on="ADXL Stream" class="WFChart (strict)"("XScale.Minimum"=w315) -> ()  [unwired: 2 in, 2 out]
                      }
                      frame #1 {
                        n137 = property on="Intan Streaming Data" class="WFChart (strict)"("XScale.Maximum"=w316) -> ()  [unwired: 2 in, 2 out]
                        n138 = property on="ADXL Stream" class="WFChart (strict)"("XScale.Maximum"=w316) -> ()  [unwired: 2 in, 2 out]
                      }
                      frame #2 {
                        n139 = property on="Intan Streaming Data" class="WFChart (strict)"("XScale.Increment"=w317) -> ()  [unwired: 2 in, 2 out]
                        n140 = property on="ADXL Stream" class="WFChart (strict)"("XScale.Increment"=w317) -> ()  [unwired: 2 in, 2 out]
                      }
                    }
                  }
                  frame 3 {
                    # "update N chans display"
                    n141 = stacked-sequence {
                      tunnel: w323 -> [w327 _ _ _ _]
                      tunnel: w319 -> [_ _ _ _ w331]
                      tunnel: w322 -> [_ _ _ w330 _]
                      tunnel: w321 -> [_ _ _ _ _]
                      tunnel: w320 -> [w325 _ _ _ _]
                      tunnel: w318 -> [_ w328 w329 _ _]
                      frame #0 {
                        n142 = Negate(x=w327) -> (-x=w326:i32)
                        n143 = Multiply(x=w325, y=w326) -> (x*y=w324:dbl)
                        n144 = property on="Intan Streaming Data" class="WFChart (strict)"("YScale.Minimum"=w324) -> ()  [unwired: 2 in, 2 out]
                      }
                      frame #1 {
                        n145 = property on="Intan Streaming Data" class="WFChart (strict)"("XScale.Offset"=w328) -> ()  [unwired: 2 in, 2 out]
                      }
                      frame #2 {
                        n146 = property on="Intan Streaming Data" class="WFChart (strict)"("XScale.Minimum"=w329) -> ()  [unwired: 2 in, 2 out]
                      }
                      frame #3 {
                        n147 = property on="Intan Streaming Data" class="WFChart (strict)"("XScale.Maximum"=w330) -> ()  [unwired: 2 in, 2 out]
                      }
                      frame #4 {
                        n148 = property on="Intan Streaming Data" class="WFChart (strict)"("XScale.Increment"=w331) -> ()  [unwired: 2 in, 2 out]
                      }
                    }
                  }
                  frame 4 {
                    # "updated offset factor"
                    n149 = stacked-sequence {
                      seq-local: [w338 _ _] -> [_ w342 _]
                      tunnel: w337 -> [_ _ _]
                      tunnel: w336 -> [_ _ _]
                      tunnel: w335 -> [_ _ _]
                      tunnel: w334 -> [w341 _ _]
                      tunnel: w333 -> [w339 _ _]
                      tunnel: w332 -> [_ _ w347]
                      frame #0 {
                        n150 = Negate(x=w341) -> (-x=w340:i32)
                        n151 = Multiply(x=w339, y=w340) -> (x*y=w338:dbl)
                        n152 = property on="Intan Streaming Data" class="WFChart (strict)"("YScale.Minimum"=w338) -> ()  [unwired: 2 in, 2 out]
                      }
                      frame #1 {
                        n153 = for {
                          N: w342 -> [_]
                          tunnel: [w345] -> w344 mode=indexing
                          i -> [w346]
                          n154 = Negate(x=w346) -> (-x=w345:i32)
                        }
                        n155 = To Double Precision Float(number=w344) -> (double precision float=w343:dbl[])
                        n156 = property on="Intan Streaming Data" class="WFChart (strict)" props=["YScale", "MarkerVals[]", "YScale", "MarkerVals[]"]("YScale.MarkerVals[]"=w343) -> ()  [unwired: 2 in, 3 out]
                      }
                      frame #2 {
                        n157 = property on="Intan Streaming Data" class="WFChart (strict)"("XScale.Increment"=w347) -> ()  [unwired: 2 in, 2 out]
                      }
                    }
                  }
                }
              }
            }
            n158 = Unbundle By Name("Filter settings") -> ("LP Filter On/Off"=w277:bool, "HP Filter On/Off"=w276:bool, "Bandstop On/Off"=w274:bool)
            n159 = Compound Arithmetic op=OR("Center Traces", w277, w276, w274) -> (w275:bool)
            n160 = case shown="True" w275 {
              tunnel: w281 -> [_ w357]
              tunnel: w279 -> [w352 w356]
              tunnel: [w352 w355] -> w269
              tunnel: "Filter settings" -> [_ w354]
              tunnel: "Center Traces" -> [_ w353]
              frame False {
              }
              frame True {
                n161 = call "Intan_filter_signals_for_display_v2.vi"("Center Traces"=w353, "input filter cluster"=w354, "Sample Rate (Hz)"=w357, "Nchan Array In [Nchans x Nsamps]"=w356) -> ("Display Signals Out [Nchans x Nsamps]"=w355:dbl[][])
              }
            }
            n162 = property on="DisplayScale (uV/div)" class="Ring (strict)"() -> ("RingText.Text"=w280:string)  [unwired: 2 in, 2 out]
            n163 = Decimal String To Number(string=w280) -> (number=w282:i32)  [unwired: 2 in, 1 out]
            n164 = call "Intan_binary_to_uV_offset_and_scale.vi"("offset spacing factor"="offset factor", "Yscale (uv/div)"=w282, "ScaledData [Nchans x Nsamps]"=w269) -> ("Nchannels"=w265:i32, "Data4Display"=w267:dbl[][])  [unwired: 1 in]
            "Intan Streaming Data" <- w267
            n165 = case shown="True" w271 {
              tunnel: w267 -> [_ w351]
              tunnel: [w348 w350] -> w272
              tunnel: w270 -> [w348 w349]
              frame False {
              }
              frame True {
                n166 = call "Intan_SaveDisplayData.vi"("2d ADCdata_array out"=w351, "aux file ref num"=w349) -> ("refnum out"=w350:refnum<file>)  [unwired: 3 in]
              }
            }
            "ADXL Stream" <- w261
          }
        }
        n167 = local read "StopLoopsMaster"() -> (w175:bool)
        "display iter" <- w195
      }
      n168 = property on="NchansInStream" class="DigNum (strict)" props=["Value"]() -> ()  [unwired: 2 in, 3 out]
      n169 = while {
        tunnel: [w360] -> w145
        tunnel: [w398] -> w148
        tunnel: w146 -> [w394]
        tunnel: "refnum in" -> [w397]
        tunnel: w147 -> [w395]
        tunnel: w144 -> [_]
        tunnel: w140 -> [w363]
        tunnel: [w367] -> w137
        tunnel: w130 -> [w358]
        i -> [w396]
        stop <- w399 stop-if-true
        w373 = T11 0 items=["no dialog", "OK message", "continue or stop message", "OK message + warnings", "continue/stop + warnings"] ("type of dialog (OK msg:1)")
        # "N data scans to read"
        # "Do we really need to slow vi loop speed here ?? JE 07 June 2019"
        # "Fs (Hz)"
        # "no warning or error = 0;\nwarning > 0 (usually harmless like buffer visa port underflow\nerror code < 0, true error encountered (e.g. visa port  premature disconnect)"
        # "READ and SAVE SERIAL DATA LOOP"
        # "monitor software ring buffer for overflow"
        # "write (append) all bytes read to binary file\nmake sure prepend is set to FALSE."
        # "unflatten data to convert from binary stream to uint16."
        # "Stop on error or if user clicks \non the stop button"
        # ">> Error Cluster >>"
        # ">> VISA Resource Name >>"
        # "read from bytes at serial port:\nCritical to set VISA I/O mode here to synchronous (else get BSOD crash)\nhttps://forums.ni.com/t5/LabVIEW/Why-do-I-get-a-blue-screen-using-USB-communication/td-p/2429322"
        n170 = Reciprocal(x=w363) -> (1/x=w377:dbl)
        n171 = Divide(x="Buffer Read Interval (ms)", y=1000.0) -> (x/y=w365:dbl)
        n172 = Multiply(x=w365, y=w363) -> (x*y=w366:dbl)
        n173 = Round Toward -Infinity(1:w366) -> (0:w362:dbl)
        "N data scans to read (VISA)" <- w362
        n174 = Multiply(x=w362, y=w377) -> (x*y=w379:dbl)
        n175 = Multiply(x=w362, y=w358) -> (x*y=w380:dbl)
        "requestBytes" <- w380
        n176 = Multiply(x=w379, y=1000.0) -> ()  [unwired: 1 out]
        n177 = VISA Read(VISA resource name=w395, byte count=w380, error in (no error)=w394) -> (VISA resource name out=w360:refnum<visa-resource-name>, read buffer=w388:string, return count=→"Nbytes VISA read":u32, error out=w375:errorcluster)
        "SerRead" <- w388
        n178 = Wait (ms)(milliseconds to wait="Buffer Read Interval (ms)") -> ()  [unwired: 1 out]
        n179 = To Unsigned Word Integer(number=i16[] []) -> (unsigned 16bit integer=w390:u16[])
        n180 = Unflatten From String(type=w390, binary string=w388, data includes array or string size? (T)=FALSE, byte order (0:big-endian, network order)="byte order") -> (value=w382:u16[])  [unwired: 1 in, 2 out]
        "binary data (from VISA read)" <- w382
        n181 = case shown="False" "Save Binary Data" {
          tunnel: [w409 w416] -> w376
          tunnel: [w408 w415] -> w398
          tunnel: w397 -> [w408 w414]
          tunnel: w375 -> [w409 w413]
          tunnel: "byte order" -> [_ w411]
          tunnel: w382 -> [_ w410]
          frame False {
          }
          frame True {
            n182 = Write to Binary File(file (use dialog)=w414, data=w410, error in=w413, 5:FALSE ("prepend array or string size? (T)"), 9:w411) -> (refnum out=w415:refnum<file>, error out=w416:errorcluster)  [unwired: 1 in, 1 out]
          }
        }
        n183 = Merge Errors(w376, w375) -> (w374:errorcluster)
        n184 = Array Size(array=w382) -> (size(s)=→"N_u16s  write to buf":i32)
        n185 = call <vilib>:"Simple Error Handler.vi"("type of dialog (OK msg:1)"=w373, "error in (no error)"=w374) -> ("code out"=w370:i32, "error out"=w371:errorcluster)  [unwired: 3 in, 3 out]
        "error code out" <- w370
        n186 = Less Than 0?(x=w370) -> (x < 0?=w368:bool)
        n187 = call-poly "Circular Buffer.vi"("Operation"=Circular_Buffer_Operations."Write", "Data In"=w382) -> ("Buffer Status"=w384:T1)  [unwired: 6 in, 3 out]
        "Buffer Status (write)" <- w384
        n188 = Equal?(x=Circular_Buffer_Status."Overflow" ("y"), y=w384) -> (x = y?=→"buffer overflow":bool)
        n189 = case shown="False" w368 {
          tunnel: w371 -> [w402 w406]
          tunnel: [FALSE TRUE] -> w369
          tunnel: [w402 w404] -> w367
          frame False {
          }
          frame True {
            n190 = call <vilib>:"Clear Errors.vi"("error in (no error)"=w406) -> ("error out"=w404:errorcluster)  [unwired: 5 in, 1 out]
            n191 = One Button Dialog(message=" stop loop, attempt graceful exit\nvisa read error") -> ()  [unwired: 1 in, 1 out]
          }
        }
        n192 = Compound Arithmetic op=OR(w369, "stop streaming") -> (w399:bool)
        "StopLoopsMaster" <- w399
        n193 = case shown="False" "stop logging" {
          tunnel: w360 -> [_ w401]
          frame False {
          }
          frame True {
            # "turns off SD logging"
            n194 = VISA Write(VISA resource name=w401, write buffer="stop logging Teensy char") -> ()  [unwired: 1 in, 3 out]
          }
        }
        "VISA read iter" <- w396
        "Save status" <- "Save Binary Data"
      }
    }
    frame #4 {
      w430 = u16 2 items=["None", "Last Bit", "TermChar"] ("Serial Settings:End Mode for Reads")
      # "There may still be some bytes waiting from last serial.write\nafter the 'p' char is sent to Teensy. Clearing the port just makes\nit more likely we see the Teensy response text response to 'p' \nby getting rid of 'extra' data bytes waiting"
      # "After user terminates acquisition (or error), need to:\n- write 'q' to Teensy to pause serial writes. Note: SPI/ADC converts + writing to SD card continues for ambulatory system\n- close VISA session\n- close LV data file\nNote we turn term char en = true so we can read out user friendly text after pausing"
      n195 = local read "Save Binary Data"() -> (w417:bool)
      n196 = case shown="True" w418 {
        tunnel: w420 -> [_ w441]
        frame False {
        }
        frame True {
          n197 = Close File(refnum=w441) -> ()  [unwired: 1 in, 2 out]
        }
      }
      n198 = property class="Serial Instr"(reference=w425, error in=w419, "TermChar En"=TRUE ("Message Based Settings:Termination Character Enable"), "ASRL End In"=w430) -> (reference out=w424:refnum<visa-resource-name>, error out=w423:errorcluster)
      n199 = case shown="True" w417 {
        tunnel: w438 -> [_ w439]
        frame False {
        }
        frame True {
          n200 = Close File(refnum=w439) -> (error out=w440:errorcluster)  [unwired: 1 in, 1 out]
          n201 = call <vilib>:"Simple Error Handler.vi"("error in (no error)"=w440) -> ()  [unwired: 4 in, 5 out]
        }
      }
      n202 = VISA Clear(VISA resource name=w424, error in (no error)=w423) -> (VISA resource name out=w422:refnum<visa-resource-name>, error out=w421:errorcluster)
      n203 = VISA Write(VISA resource name=w422, write buffer="stop serial stream (Teensy char)", error in (no error)=w421) -> (VISA resource name out=w433:refnum<visa-resource-name>, error out=w432:errorcluster)  [unwired: 1 out]
      n204 = VISA Read(VISA resource name=w433, byte count=u32 20000, error in (no error)=w432) -> (VISA resource name out=w429:refnum<visa-resource-name>, read buffer=→"Text response":string, error out=w427:errorcluster)  [unwired: 1 out]
      n205 = VISA Clear(VISA resource name=w429, error in (no error)=w427) -> (VISA resource name out=w428:refnum<visa-resource-name>, error out=w426:errorcluster)
      n206 = VISA Close(VISA resource name=w428, error in (no error)=w426) -> (error out=→"error out":errorcluster)
    }
  }
